vi "Configure Power Measurement List Single Index Repetition.vi"(7 "Repetitions (1)":i32=1, 8 "error in (no error)":errorcluster, 9 "Index (0)":i32, 10 "Instance (1)":i32=1, 11 "VISA resource name":refnum<visa-resource-name>) -> (0 "error out":errorcluster, 3 "VISA resource name out":refnum<visa-resource-name>)   [LabVIEW 2020, in "Rohde&Schwarz CMXP GPRF.lvlib"]
doc: "Defines the \"Index Repetion\" of a selected frequency/level step.\n\nAttribute:\nRSCMXPGPRF_ATTR_POWER_MEASUREMENT_LIST_SINGLE_INDEX_REPETITION\n\nRemote-control command:\nCONFigure:GPRF:MEAS<i>:POWer:LIST:IREPetition"
uses:
  <instrlib>/Rohde&Schwarz CMXP GPRF/Rohde&Schwarz CMXP GPRF.lvlib
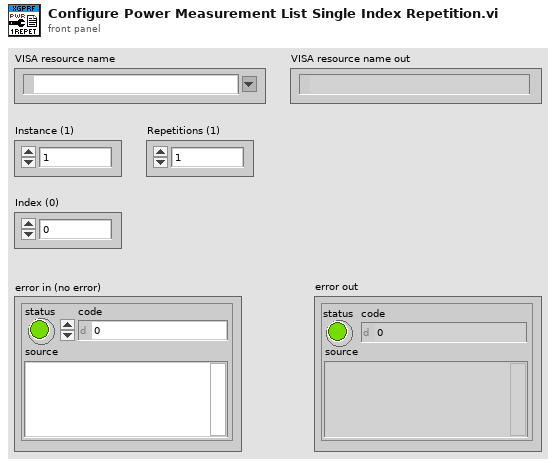
[diagram p1: front panel]
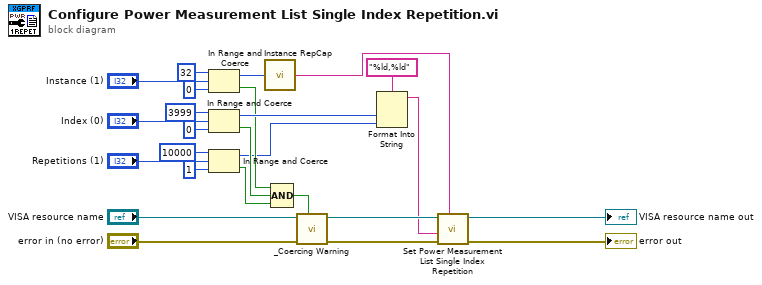
[diagram p0: block diagram]
diagram:
  n1 = In Range and Coerce(upper limit=32, x="Instance (1)", lower limit=0) -> (coerced(x)=w11:i32, In Range?=w3:bool)
  n2 = In Range and Coerce(upper limit=3999, x="Index (0)", lower limit=0) -> (coerced(x)=w12:i32, In Range?=w4:bool)
  n3 = In Range and Coerce(upper limit=10000, x="Repetitions (1)", lower limit=1) -> (coerced(x)=w2:i32, In Range?=w5:bool)
  n4 = call <instrlib>:"Instance RepCap.vi"("Instance in"=w11) -> ("Instance out"=w6:string)
  n5 = Compound Arithmetic op=AND(w3, w4, w5) -> (w20:bool)
  n6 = call <instrlib>:"_Coercing Warning.vi"("In Range?"=w20, "error in (no error)"="error in (no error)", "VISA resource name"="VISA resource name") -> ("error out"=w10:errorcluster, "VISA resource name out"=w9:refnum<visa-resource-name>)  [unwired: 7 in]
  n7 = Format Into String(format string="%ld,%ld", w12, w2) -> (resulting string=w1:string)  [unwired: 2 in, 1 out]
  n8 = call "Set Power Measurement List Single Index Repetition"("Repeated Capabilities"=w6, "error in (no error)"=w10, "Power Measurement List Single Index Repetition ()"=w1, "instrument handle"=w9) -> ("error out"=→"error out":errorcluster, "instrument handle out"=→"VISA resource name out":refnum<visa-resource-name>)  [unwired: 6 in]
